vi "bytestream to data.vi"(7 "big endian?":bool, 9 "specifications":T1[](array[typedef]), 10 "bytestream":u8[](array[numeric]), 11 "allocation":T3) -> (3 "data table":T3)   [LabVIEW 2013, in "EthernetIP runtime.lvclass"]
uses:
  EthernetIP runtime.lvclass
  <vilib>/NI/Tag Bus/table/data table.ctl
  conversion specification.ctl
  <vilib>/NI/Tag Bus/tag/Data Type.ctl
  <vilib>/NI/Tag Bus/table/data polymorphs/write one/write Double.vi
  <vilib>/NI/Tag Bus/table/data polymorphs/write one/write Single.vi
  <vilib>/NI/Tag Bus/table/data polymorphs/write one/write I64.vi
  <vilib>/NI/Tag Bus/table/data polymorphs/write one/write U64.vi
  <vilib>/NI/Tag Bus/table/data polymorphs/write one/write I32.vi
  <vilib>/NI/Tag Bus/table/data polymorphs/write one/write U32.vi
  <vilib>/NI/Tag Bus/table/data polymorphs/write one/write I16.vi
  <vilib>/NI/Tag Bus/table/data polymorphs/write one/write U16.vi
  <vilib>/NI/Tag Bus/table/data polymorphs/write one/write I8.vi
  <vilib>/NI/Tag Bus/table/data polymorphs/write one/write U8.vi
  <vilib>/NI/Tag Bus/table/data polymorphs/write one/write Boolean.vi
  <vilib>/NI/Tag Bus/table/data polymorphs/write one/write Array of I8.vi
  <vilib>/NI/Tag Bus/table/data polymorphs/write one/write Array of U8.vi
  <vilib>/NI/Tag Bus/table/data polymorphs/write one/write Array of U64.vi
  <vilib>/NI/Tag Bus/table/data polymorphs/write one/write Array of I64.vi
  <vilib>/NI/Tag Bus/table/data polymorphs/write one/write Array of Double.vi
  <vilib>/NI/Tag Bus/table/data polymorphs/write one/write Array of U32.vi
  <vilib>/NI/Tag Bus/table/data polymorphs/write one/write Array of Single.vi
  <vilib>/NI/Tag Bus/table/data polymorphs/write one/write Array of I32.vi
  <vilib>/NI/Tag Bus/table/data polymorphs/write one/write Array of I16.vi
  <vilib>/NI/Tag Bus/table/data polymorphs/write one/write Array of U16.vi
  <vilib>/NI/Tag Bus/table/data table.lvlib
  <vilib>/NI/Tag Bus/tag/tag descriptor.lvclass
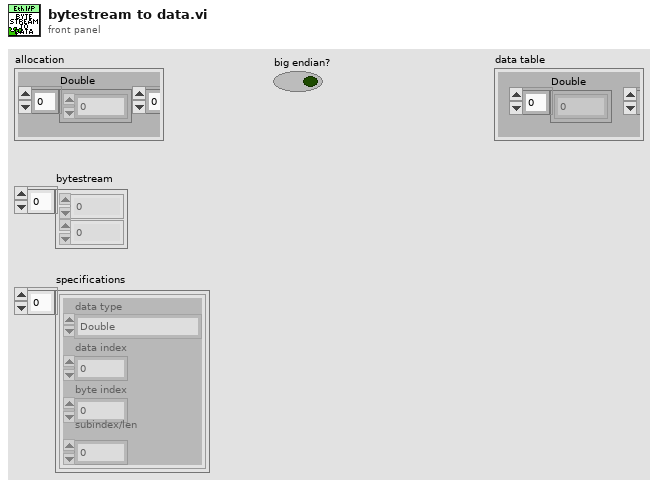
[diagram p1: front panel]
types:
  T1 = typedef "EthernetIP runtime.lvclass/conversion specification.ctl" = cluster{"data type":T2, "data index":i32, "byte index":i32, "subindex/len":i32}
  T2 = typedef "tag bus.lvlib/tag descriptor.lvclass/Data Type.ctl" = enum16{"Double", "Single", "I64", "I32", "I16", "I8", "U64", "U32", "U16", "U8", "Boolean", "String", "Array of Double", "Array of Single", "Array of I64", "Array of I32", "Array of I16", "Array of I8", "Array of U64", "Array of U32", "Array of U16", "Array of U8", "Array of Boolean", "Array of String"}
  T3 = typedef "tag bus.lvlib/data table.lvlib/data table.ctl" = cluster{"Double":dbl[], "Single":sgl[], "I64":i64[], "I32":i32[], "I16":i16[], "I8":i8[], "U64":u64[], "U32":u32[], "U16":u16[], "U8":u8[], "Boolean":bool[], "String":string[], "Array of Double":cluster{"DBL Array":dbl[]}[], "Array of Single":cluster{"SGL Array":sgl[]}[], "Array of I64":cluster{"I64 Array":i64[]}[], "Array of I32":cluster{"I32 Array":i32[]}[], "Array of I16":cluster{"I16 Array":i16[]}[], "Array of I8":cluster{"I8 Array":i8[]}[], "Array of U64":cluster{"U64 Array":u64[]}[], "Array of U32":cluster{"U32 Array":u32[]}[], "Array of U16":cluster{"U16 Array":u16[]}[], "Array of U8":cluster{"U8 Array":u8[]}[], "Array of Boolean":cluster{"Boolean Array":bool[]}[], "Array of String":cluster{"String Array":string[]}[]}
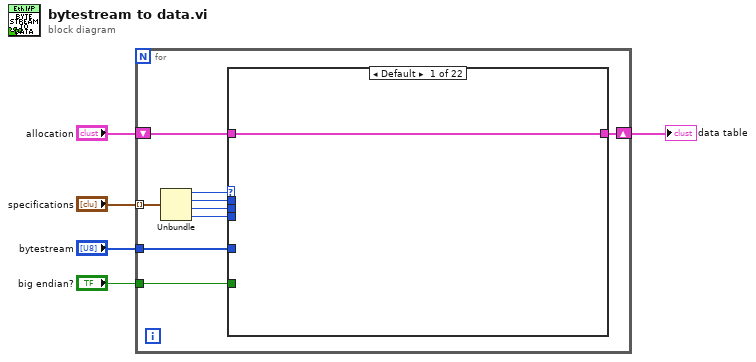
[diagram p0: block diagram]
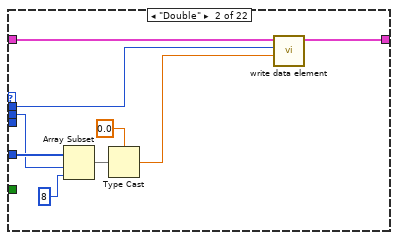
[diagram p2: hidden frame]
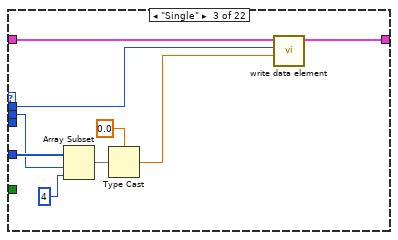
[diagram p3: hidden frame]
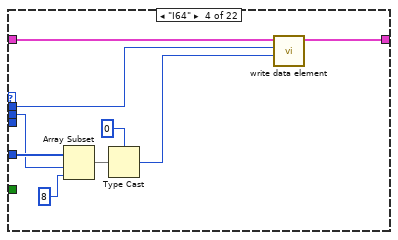
[diagram p4: hidden frame]
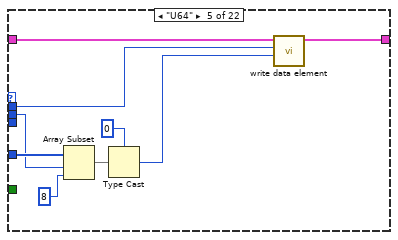
[diagram p5: hidden frame]
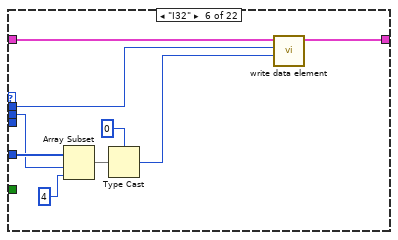
[diagram p6: hidden frame]
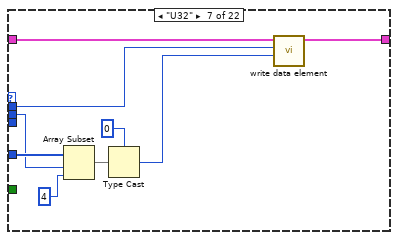
[diagram p7: hidden frame]
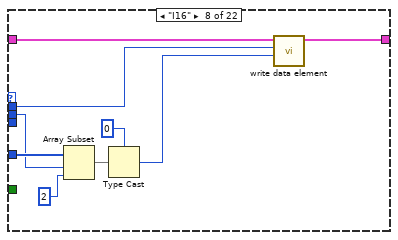
[diagram p8: hidden frame]
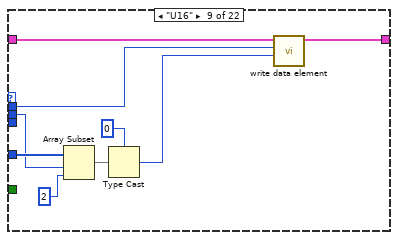
[diagram p9: hidden frame]
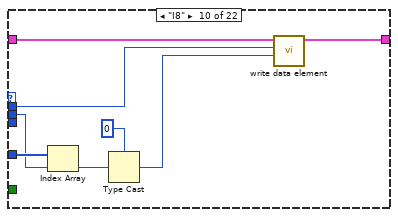
[diagram p10: hidden frame]
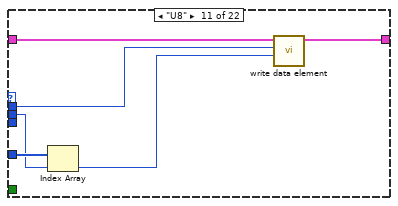
[diagram p11: hidden frame]
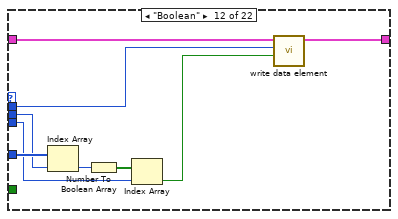
[diagram p12: hidden frame]
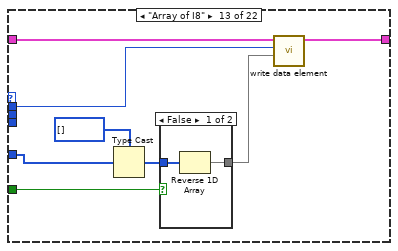
[diagram p13: hidden frame]
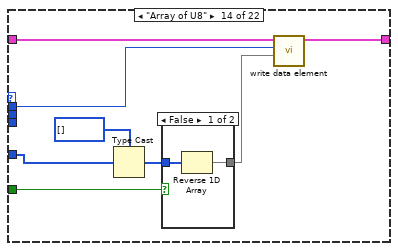
[diagram p15: hidden frame]
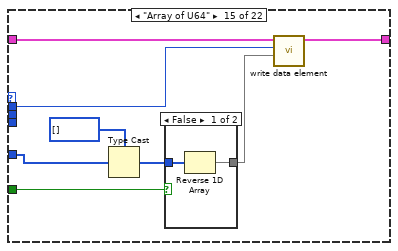
[diagram p17: hidden frame]
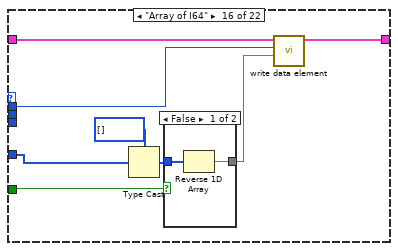
[diagram p19: hidden frame]
diagram:
  n1 = for {
    shift-right: [w11] -> w4
    shift-left: "allocation" -> [w12]
    tunnel: "bytestream" -> [w10]
    tunnel: "specifications" -> [w14] mode=indexing
    tunnel: "big endian?" -> [w6]
    n2 = Unbundle(w14) -> ("data type"=w13:T2, "data index"=w9:i32, "byte index"=w7:i32, "subindex/len"=w8:i32)
    n3 = case shown="Default" w13 {
      tunnel: w12 -> [w15 w24 w33 w42 w51 w60 w69 w78 w87 w95 w101 w110 w118 w129 w140 w151 w162 w173 w184 w195 w206 w217]
      tunnel: [w15 w23 w32 w41 w50 w59 w68 w77 w86 w94 w100 w109 w117 w128 w139 w150 w161 w172 w183 w194 w205 w216] -> w11
      tunnel: w7 -> [_ w20 w29 w38 w47 w56 w65 w74 w83 w92 w98 w107 _ _ _ _ _ _ _ _ _ _]
      tunnel: w10 -> [_ w22 w31 w40 w49 w58 w67 w76 w85 w93 w99 w108 w115 w126 w137 w148 w159 w170 w181 w192 w203 w214]
      tunnel: w9 -> [_ w19 w28 w37 w46 w55 w64 w73 w82 w91 w97 w106 w116 w127 w138 w149 w160 w171 w182 w193 w204 w215]
      tunnel: w8 -> [_ _ _ _ _ _ _ _ _ _ _ w102 _ _ _ _ _ _ _ _ _ _]
      tunnel: w6 -> [_ _ _ _ _ _ _ _ _ _ _ _ w113 w122 w133 w144 w156 w167 w178 w189 w200 w210]
      frame Default {
      }
      frame "Double" {
        n4 = Array Subset(array=w22, index=w20, length=8 ("x")) -> (w18:u8[])
        n5 = Type Cast(type=0.0, x=w18) -> (*(type *) &x=w16:dbl)
        n6 = call-poly <vilib>:"write data element.vi"("value"=w16, "index"=w19, "data table in"=w24) -> ("data table out"=w23:T3)  [unwired: 8 in]
      }
      frame "Single" {
        n7 = Array Subset(array=w31, index=w29, length=4 ("x")) -> (w27:u8[])
        n8 = Type Cast(type=sgl 0.0, x=w27) -> (*(type *) &x=w25:sgl)
        n9 = call-poly <vilib>:"write data element.vi"("value"=w25, "index"=w28, "data table in"=w33) -> ("data table out"=w32:T3)  [unwired: 8 in]
      }
      frame "I64" {
        n10 = Array Subset(array=w40, index=w38, length=8 ("x")) -> (w36:u8[])
        n11 = Type Cast(type=i64 0, x=w36) -> (*(type *) &x=w34:i64)
        n12 = call-poly <vilib>:"write data element.vi"("value"=w34, "index"=w37, "data table in"=w42) -> ("data table out"=w41:T3)  [unwired: 8 in]
      }
      frame "U64" {
        n13 = Array Subset(array=w49, index=w47, length=8 ("x")) -> (w45:u8[])
        n14 = Type Cast(type=u64 0, x=w45) -> (*(type *) &x=w43:u64)
        n15 = call-poly <vilib>:"write data element.vi"("value"=w43, "index"=w46, "data table in"=w51) -> ("data table out"=w50:T3)  [unwired: 8 in]
      }
      frame "I32" {
        n16 = Array Subset(array=w58, index=w56, length=4 ("x")) -> (w54:u8[])
        n17 = Type Cast(type=0, x=w54) -> (*(type *) &x=w52:i32)
        n18 = call-poly <vilib>:"write data element.vi"("value"=w52, "index"=w55, "data table in"=w60) -> ("data table out"=w59:T3)  [unwired: 8 in]
      }
      frame "U32" {
        n19 = Array Subset(array=w67, index=w65, length=4 ("x")) -> (w63:u8[])
        n20 = Type Cast(type=u32 0, x=w63) -> (*(type *) &x=w61:u32)
        n21 = call-poly <vilib>:"write data element.vi"("value"=w61, "index"=w64, "data table in"=w69) -> ("data table out"=w68:T3)  [unwired: 8 in]
      }
      frame "I16" {
        n22 = Array Subset(array=w76, index=w74, length=2 ("x")) -> (w72:u8[])
        n23 = Type Cast(type=i16 0, x=w72) -> (*(type *) &x=w70:i16)
        n24 = call-poly <vilib>:"write data element.vi"("value"=w70, "index"=w73, "data table in"=w78) -> ("data table out"=w77:T3)  [unwired: 8 in]
      }
      frame "U16" {
        n25 = Array Subset(array=w85, index=w83, length=2 ("x")) -> (w81:u8[])
        n26 = Type Cast(type=u16 0, x=w81) -> (*(type *) &x=w79:u16)
        n27 = call-poly <vilib>:"write data element.vi"("value"=w79, "index"=w82, "data table in"=w87) -> ("data table out"=w86:T3)  [unwired: 8 in]
      }
      frame "I8" {
        n28 = Index Array(array=w93, index=w92) -> (element=w90:u8)
        n29 = Type Cast(type=i8 0, x=w90) -> (*(type *) &x=w88:i8)
        n30 = call-poly <vilib>:"write data element.vi"("value"=w88, "index"=w91, "data table in"=w95) -> ("data table out"=w94:T3)  [unwired: 8 in]
      }
      frame "U8" {
        n31 = Index Array(array=w99, index=w98) -> (element=w96:u8)
        n32 = call-poly <vilib>:"write data element.vi"("value"=w96, "index"=w97, "data table in"=w101) -> ("data table out"=w100:T3)  [unwired: 8 in]
      }
      frame "Boolean" {
        n33 = Index Array(array=w108, index=w107) -> (element=w105:u8)
        n34 = Number To Boolean Array(number=w105) -> (Boolean array=w104:bool[])
        n35 = Index Array(array=w104, index=w102) -> (element=w103:bool)
        n36 = call-poly <vilib>:"write data element.vi"("value"=w103, "index"=w106, "data table in"=w110) -> ("data table out"=w109:T3)  [unwired: 8 in]
      }
      frame "Array of I8" {
        n37 = Type Cast(type=i8[] [] ("subarray"), x=w115) -> (*(type *) &x=w112:i8[])
        n38 = case shown="False" w113 {
          tunnel: w112 -> [w120 w121]
          tunnel: [w119 w121] -> w111
          frame False {
            n39 = Reverse 1D Array(array=w120) -> (reversed array=w119:i8[])
          }
          frame True {
          }
        }
        n40 = call-poly <vilib>:"write data element.vi"("value"=w111, "index"=w116, "data table in"=w118) -> ("data table out"=w117:T3)  [unwired: 8 in]
      }
      frame "Array of U8" {
        n41 = Type Cast(type=u8[] [] ("subarray"), x=w126) -> (*(type *) &x=w124:u8[])
        n42 = case shown="False" w122 {
          tunnel: w124 -> [w131 w132]
          tunnel: [w130 w132] -> w123
          frame False {
            n43 = Reverse 1D Array(array=w131) -> (reversed array=w130:u8[])
          }
          frame True {
          }
        }
        n44 = call-poly <vilib>:"write data element.vi"("value"=w123, "index"=w127, "data table in"=w129) -> ("data table out"=w128:T3)  [unwired: 8 in]
      }
      frame "Array of U64" {
        n45 = Type Cast(type=u64[] [] ("subarray"), x=w137) -> (*(type *) &x=w135:u64[])
        n46 = case shown="False" w133 {
          tunnel: w135 -> [w142 w143]
          tunnel: [w141 w143] -> w134
          frame False {
            n47 = Reverse 1D Array(array=w142) -> (reversed array=w141:u64[])
          }
          frame True {
          }
        }
        n48 = call-poly <vilib>:"write data element.vi"("value"=w134, "index"=w138, "data table in"=w140) -> ("data table out"=w139:T3)  [unwired: 8 in]
      }
      frame "Array of I64" {
        n49 = Type Cast(type=i64[] [] ("subarray"), x=w148) -> (*(type *) &x=w146:i64[])
        n50 = case shown="False" w144 {
          tunnel: w146 -> [w153 w154]
          tunnel: [w152 w154] -> w145
          frame False {
            n51 = Reverse 1D Array(array=w153) -> (reversed array=w152:i64[])
          }
          frame True {
          }
        }
        n52 = call-poly <vilib>:"write data element.vi"("value"=w145, "index"=w149, "data table in"=w151) -> ("data table out"=w150:T3)  [unwired: 8 in]
      }
      frame "Array of Double" {
        n53 = Type Cast(type=dbl[] [] ("subarray"), x=w159) -> (*(type *) &x=w157:dbl[])
        n54 = case shown="False" w156 {
          tunnel: w157 -> [w164 w165]
          tunnel: [w163 w165] -> w155
          frame False {
            n55 = Reverse 1D Array(array=w164) -> (reversed array=w163:dbl[])
          }
          frame True {
          }
        }
        n56 = call-poly <vilib>:"write data element.vi"("value"=w155, "index"=w160, "data table in"=w162) -> ("data table out"=w161:T3)  [unwired: 8 in]
      }
      frame "Array of U32" {
        n57 = Type Cast(type=u32[] [] ("subarray"), x=w170) -> (*(type *) &x=w168:u32[])
        n58 = case shown="False" w167 {
          tunnel: w168 -> [w175 w176]
          tunnel: [w174 w176] -> w166
          frame False {
            n59 = Reverse 1D Array(array=w175) -> (reversed array=w174:u32[])
          }
          frame True {
          }
        }
        n60 = call-poly <vilib>:"write data element.vi"("value"=w166, "index"=w171, "data table in"=w173) -> ("data table out"=w172:T3)  [unwired: 8 in]
      }
      frame "Array of Single" {
        n61 = Type Cast(type=sgl[] [] ("subarray"), x=w181) -> (*(type *) &x=w179:sgl[])
        n62 = case shown="False" w178 {
          tunnel: w179 -> [w186 w187]
          tunnel: [w185 w187] -> w177
          frame False {
            n63 = Reverse 1D Array(array=w186) -> (reversed array=w185:sgl[])
          }
          frame True {
          }
        }
        n64 = call-poly <vilib>:"write data element.vi"("value"=w177, "index"=w182, "data table in"=w184) -> ("data table out"=w183:T3)  [unwired: 8 in]
      }
      frame "Array of I32" {
        n65 = Type Cast(type=i32[] [] ("subarray"), x=w192) -> (*(type *) &x=w190:i32[])
        n66 = case shown="False" w189 {
          tunnel: w190 -> [w197 w198]
          tunnel: [w196 w198] -> w188
          frame False {
            n67 = Reverse 1D Array(array=w197) -> (reversed array=w196:i32[])
          }
          frame True {
          }
        }
        n68 = call-poly <vilib>:"write data element.vi"("value"=w188, "index"=w193, "data table in"=w195) -> ("data table out"=w194:T3)  [unwired: 8 in]
      }
      frame "Array of I16" {
        n69 = Type Cast(type=i16[] [] ("subarray"), x=w203) -> (*(type *) &x=w201:i16[])
        n70 = case shown="False" w200 {
          tunnel: w201 -> [w208 w209]
          tunnel: [w207 w209] -> w199
          frame False {
            n71 = Reverse 1D Array(array=w208) -> (reversed array=w207:i16[])
          }
          frame True {
          }
        }
        n72 = call-poly <vilib>:"write data element.vi"("value"=w199, "index"=w204, "data table in"=w206) -> ("data table out"=w205:T3)  [unwired: 8 in]
      }
      frame "Array of U16" {
        n73 = Type Cast(type=u16[] [] ("subarray"), x=w214) -> (*(type *) &x=w212:u16[])
        n74 = case shown="False" w210 {
          tunnel: w212 -> [w219 w220]
          tunnel: [w218 w220] -> w211
          frame False {
            n75 = Reverse 1D Array(array=w219) -> (reversed array=w218:u16[])
          }
          frame True {
          }
        }
        n76 = call-poly <vilib>:"write data element.vi"("value"=w211, "index"=w215, "data table in"=w217) -> ("data table out"=w216:T3)  [unwired: 8 in]
      }
    }
  }
  "data table" <- w4
